vi "AutoSetSteerAngle.vi"(11 "Angle":dbl) -> ()   [LabVIEW 2014]
uses:
  Automated Tasks/AutomationGlobals.vi
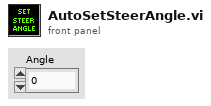
[diagram p1: front panel]
types:
  T1 = typedef "WPI_MotorControlDeviceRef.ctl" = cluster{"DeviceStatus":errorcluster, "Type":T2, "PWM":cluster{"Controller":T3, "PWM Channel":T4, "DeadBand":T5}, "CAN":cluster{"Device Number":u8, "Control Mode":T6, "Semaphore":T7, "Max Vout":dbl, "TalonSRX Control Mode":T8}, "Invert":bool, "TransformRef":T9, "InvTransformRef":T9}
  T2 = typedef "WPI_MotorControlType.ctl" = enum16{"PWM", "CAN", "CANTalonSRX"}
  T3 = typedef "FPGA_TypedefDigitalModule.ctl" = enum16{"Controller 1"}
  T4 = typedef "FPGA_DIOPWMChannel.ctl" = enum8{"PWM 0", "PWM 1", "PWM 2", "PWM 3", "PWM 4", "PWM 5", "PWM 6", "PWM 7", "PWM 8", "PWM 9", "PWM MXP 0", "PWM MXP 1", "PWM MXP 2", "PWM MXP 3", "PWM MXP 4", "PWM MXP 5", "PWM MXP 6", "PWM MXP 7", "PWM MXP 8", "PWM MXP 9", "Invalid"}
  T5 = typedef "WPI_PWMDeadband.ctl" = cluster{"Name":string, "maxPositivePwm":i32, "minPositivePwm":i32, "centerPwm":i32, "maxNegativePwm":i32, "minNegativePwm":i32, "angularRange":u16}
  T6 = typedef "WPI_CANJaguar_ControlMode.ctl" = enum8{"Percent VBus", "Current", "Speed", "Position", "Voltage"}
  T7 = typedef "Semaphore RefNum" = refnum<k1>
  T8 = typedef "WPI_CANTalonSRX_APIControlMode.ctl" = enum8{"Percent VBus", "Speed", "Position", "Slave", "Unchanged / Invalid"}
  T9 = typedef "WPI_PWMTransform_ConPane.ctl" = refnum<vi>
  T10 = typedef "WPI_CANTalonSRX_GlobalStatus.ctl" = cluster{"Applied Throttle":dbl, "Module Enabled":bool, "CAN Error":errorcluster, "Closed Loop Error":dbl, "Forward Limit Switch Closed":bool, "Reverse Limit Switch Closed":bool, "Sensor Position":dbl, "Sensor Velocity":dbl, "Current":dbl, "Sticky Fault - Over Temp":bool, "Sticky Fault - Under Voltage":bool, "Sticky Fault - Forward Limit":bool, "Sticky Fault - Reverse Limit":bool, "Sticky Fault - Forward Soft Limit":bool, "Sticky Fault - Reverse Soft Limit":bool, "Brake is Enabled":bool, "Encoder Position":dbl, "Encoder Velocity":dbl, "Encoder Index Count":dbl, "Encoder A Pin State":bool, "Encoder B Pin State":bool, "Encoder Index Pin State":bool, "Analog In":dbl, "Analog In Velocity":dbl, "Temperature (C)":dbl, "Battery Voltage":dbl}
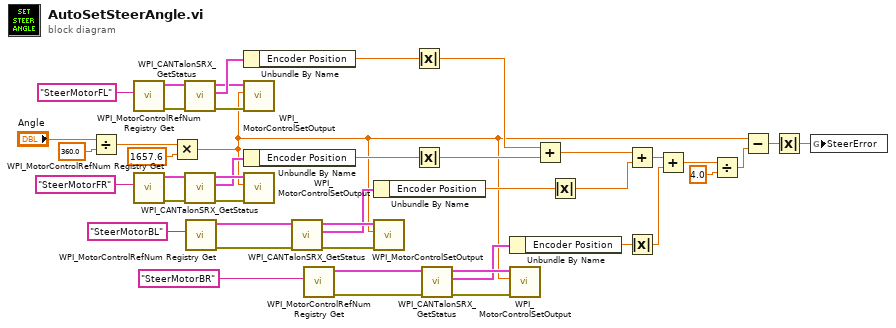
[diagram p0: block diagram]
diagram:
  n1 = Divide(x="Angle", y=360.0) -> (x/y=w2:dbl)
  n2 = call <vilib>:"WPI_MotorControlRefNum Registry Get.vi"("refnum name"="SteerMotorFL") -> ("error out"=w37:errorcluster, "MotorControlDevRef"=w36:T1)  [unwired: 9 in]
  n3 = call <vilib>:"WPI_MotorControlRefNum Registry Get.vi"("refnum name"="SteerMotorFR") -> ("error out"=w39:errorcluster, "MotorControlDevRef"=w38:T1)  [unwired: 9 in]
  n4 = Multiply(x=w2, y=1657.6 ("Angle")) -> (x*y=w7:dbl)
  n5 = call <vilib>:"WPI_CANTalonSRX_GetStatus.vi"("error in (no error)"=w37, "CAN Talon SRX Ref"=w36) -> ("error out"=w31:errorcluster, "Talon SRX Status"=w30:T10, "CAN Talon SRX Ref Out"=w20:T1)  [unwired: 7 in]
  n6 = call <vilib>:"WPI_CANTalonSRX_GetStatus.vi"("error in (no error)"=w39, "CAN Talon SRX Ref"=w38) -> ("error out"=w28:errorcluster, "Talon SRX Status"=w27:T10, "CAN Talon SRX Ref Out"=w29:T1)  [unwired: 7 in]
  n7 = call <vilib>:"WPI_MotorControlRefNum Registry Get.vi"("refnum name"="SteerMotorBL") -> ("error out"=w41:errorcluster, "MotorControlDevRef"=w40:T1)  [unwired: 9 in]
  n8 = Unbundle By Name(w30) -> ("Encoder Position"=w19:dbl)
  n9 = call <vilib>:"WPI_MotorControlSetOutput.vi"("error in (no error)"=w31, "Output"=w7, "MotorControlDevRef"=w20) -> ()  [unwired: 6 in, 3 out]
  n10 = Unbundle By Name(w27) -> ("Encoder Position"=w18:dbl)
  n11 = call <vilib>:"WPI_MotorControlSetOutput.vi"("error in (no error)"=w28, "Output"=w7, "MotorControlDevRef"=w29) -> ()  [unwired: 6 in, 3 out]
  n12 = call <vilib>:"WPI_CANTalonSRX_GetStatus.vi"("error in (no error)"=w41, "CAN Talon SRX Ref"=w40) -> ("error out"=w25:errorcluster, "Talon SRX Status"=w24:T10, "CAN Talon SRX Ref Out"=w26:T1)  [unwired: 7 in]
  n13 = call <vilib>:"WPI_MotorControlRefNum Registry Get.vi"("refnum name"="SteerMotorBR") -> ("error out"=w43:errorcluster, "MotorControlDevRef"=w42:T1)  [unwired: 9 in]
  n14 = Unbundle By Name(w24) -> ("Encoder Position"=w16:dbl)
  n15 = call <vilib>:"WPI_MotorControlSetOutput.vi"("error in (no error)"=w25, "Output"=w7, "MotorControlDevRef"=w26) -> ()  [unwired: 6 in, 3 out]
  n16 = Absolute Value(x=w19) -> (abs(x)=w11:dbl)
  n17 = Absolute Value(x=w18) -> (abs(x)=w10:dbl)
  n18 = call <vilib>:"WPI_CANTalonSRX_GetStatus.vi"("error in (no error)"=w43, "CAN Talon SRX Ref"=w42) -> ("error out"=w22:errorcluster, "Talon SRX Status"=w21:T10, "CAN Talon SRX Ref Out"=w23:T1)  [unwired: 7 in]
  n19 = Unbundle By Name(w21) -> ("Encoder Position"=w14:dbl)
  n20 = call <vilib>:"WPI_MotorControlSetOutput.vi"("error in (no error)"=w22, "Output"=w7, "MotorControlDevRef"=w23) -> ()  [unwired: 6 in, 3 out]
  n21 = Add(x=w11, y=w10) -> (x+y=w17:dbl)
  n22 = Absolute Value(x=w16) -> (abs(x)=w9:dbl)
  n23 = Add(x=w17, y=w9) -> (x+y=w15:dbl)
  n24 = Absolute Value(x=w14) -> (abs(x)=w8:dbl)
  n25 = Add(x=w15, y=w8) -> (x+y=w13:dbl)
  n26 = Divide(x=w13, y=4.0) -> (x/y=w6:dbl)
  n27 = Subtract(x=w7, y=w6) -> (x-y=w5:dbl)
  n28 = Absolute Value(x=w5) -> (abs(x)=w4:dbl)
  n29 = global write "AutomationGlobals.vi" "SteerError"(w4) -> ()
